vi "CreateIntegerArray.vi"() -> ()   [LabVIEW 2014]
uses:
  <vilib>/imath/engines/lvmath2/RunTimeEngine/Managers/WorkSpace/UID Generator.vi
  <vilib>/imath/engines/lvmath2/RunTimeEngine/RunTimeType/NIMS_RunTimeType_From StrictType (excl LVString).vi
  <instcachedir>/0/NIMS_RunTimeType_From StrictType (excl LVString)_15A5391EEA9C4AACB9955AC755B83D29.lvgen/NIMS_RunTimeType_From StrictType (excl LVString)_15A5391EEA9C4AACB9955AC755B83D29_000.vi
  <vilib>/imath/engines/lvmath2/RunTimeEngine/LocalVariableDefStatement/MC_LocalVariableDefStatement_Display.vi
  <vilib>/imath/engines/lvmath2/RunTimeSupport/NIMS_Complex To Real.vi
  <instcachedir>/0/NIMS_Complex To Real_CFEFC05793354143908F7AF8F5FCAA9D.lvgen/NIMS_Complex To Real_CFEFC05793354143908F7AF8F5FCAA9D_001.vi
  <vilib>/imath/engines/lvmath2/RunTimeEngine/BuiltInFunctions/logramp/NIMS_logramp.vi
  <vilib>/imath/engines/lvmath2/RunTimeEngine/ErrorHandling/NIMS_Create Error From Enums.vi
  <vilib>/imath/engines/lvmath2/RunTimeEngine/Managers/SymbolTable/Clear UID.vi
  <vilib>/imath/engines/lvmath2/RunTimeEngine/NodeEndStatement/NIMS_NodeEndStatement_Output.vi
  <instcachedir>/0/NIMS_NodeEndStatement_Output_53EC0D466D134D7ABD903AC30B43404B.lvgen/NIMS_NodeEndStatement_Output_53EC0D466D134D7ABD903AC30B43404B_005.vi
  <vilib>/imath/engines/lvmath2/RunTimeEngine/ErrorHandling/NIMS_Finalize Error.vi
  <vilib>/imath/engines/lvmath2/RunTimeEngine/BuiltInFunctions/linramp/NIMS_linramp.vi
  <vilib>/imath/engines/lvmath2/RunTimeEngine/Managers/SymbolTable/NIMS_WorkSpace.lvlib
panel:
  out "Out":dbl[](array[numeric])
  in  "Spacing":enum16{"Logarithmic", "Linear"}(ring)
  in  "# of Points":dbl
  in  "Maximum":dbl
  in  "Minimum":dbl
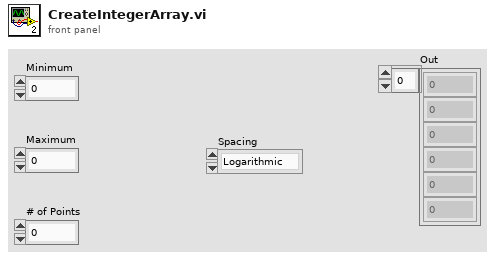
[diagram p1: front panel]
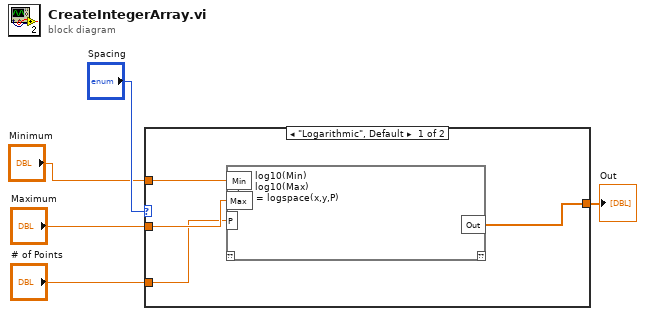
[diagram p0: block diagram]
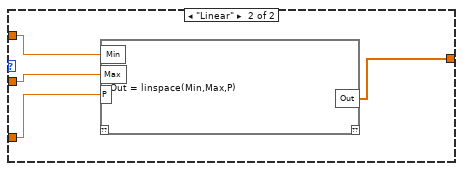
[diagram p2: hidden frame]
diagram:
  n1 = case shown="\"Logarithmic\", Default" "Spacing" {
    tunnel: "Minimum" -> [w9 w103]
    tunnel: "Maximum" -> [w8 w102]
    tunnel: "# of Points" -> [w7 w101]
    tunnel: [w6 w100] -> w1
    frame "Logarithmic", Default {
      n2 = mathscript code="x = log10(Min)\ny = log10(Max)\nOut = logspace(x,y,P)"("Min"=w9, "Max"=w8, "P"=w7) -> ("Out"=w6:dbl[])  [unwired: 1 in, 1 out]
    }
    frame "Linear" {
      n3 = mathscript code="Out = linspace(Min,Max,P)"("Min"=w103, "Max"=w102, "P"=w101) -> ("Out"=w100:dbl[])  [unwired: 1 in, 1 out]
    }
  }
  "Out" <- w1
